vi "MakePath.vi"(9 "Strings []":string[](array[string]), 10 "ChannelToCompensate":i32, 11 "TimeTraceSaveLocation":path) -> (2 "Numeric Control":i32, 3 "appended path":path)   [LabVIEW 2011]
uses:
  Globals/Meas_global.vi
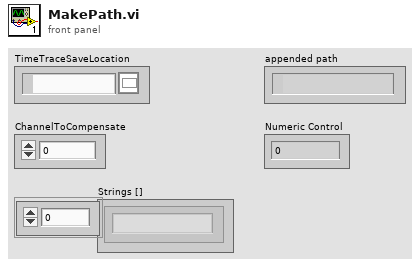
[diagram p1: front panel]
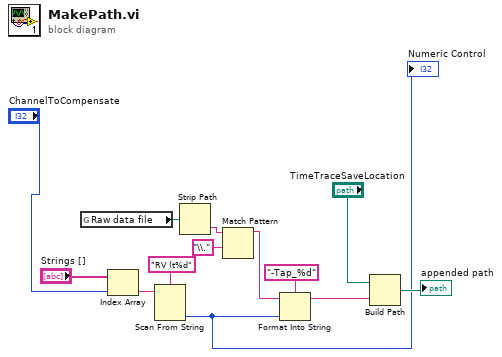
[diagram p0: block diagram]
diagram:
  n1 = global read "Meas_global.vi" "Raw data file"() -> (w4:path)
  n2 = Index Array(array="Strings []", index="ChannelToCompensate") -> (element=w2:string)
  n3 = Scan From String(format string="RV (t%d", input string=w2) -> (output 1=w10:i32)  [unwired: 3 in, 3 out]
  "Numeric Control" <- w10
  n4 = Strip Path(path=w4) -> (name=w5:string)  [unwired: 1 out]
  n5 = Match Pattern(string=w5, regular expression="\\.") -> (before substring=w7:string)  [unwired: 1 in, 3 out]
  n6 = Format Into String(format string="-Tap_%d", initial string=w7, w10) -> (resulting string=w12:string)  [unwired: 1 in, 1 out]
  n7 = Build Path(base path="TimeTraceSaveLocation", name or relative path=w12) -> (appended path=→"appended path":path)
